vi "set_status_string.vi"(8 "error in":errorcluster, 9 "new line?":bool=TRUE, 10 "status string in":string, 11 "controls array":refnum<vi>[](array[refnum])) -> (0 "error out":errorcluster, 3 "controls array out":refnum<vi>[](array[refnum]))   [LabVIEW 2019]
panel:
  out "output string":string
  # "SET STATUS STRING"
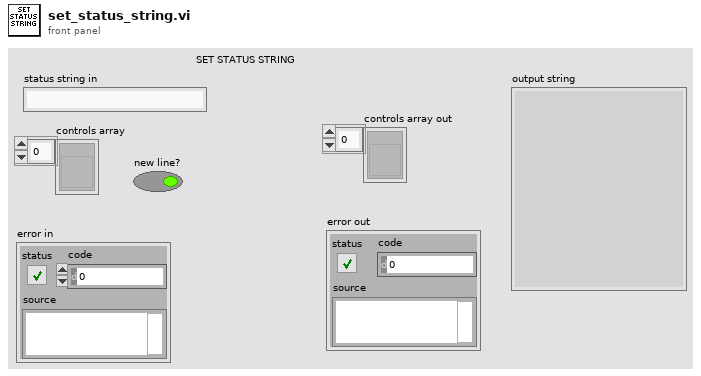
[diagram p1: front panel]
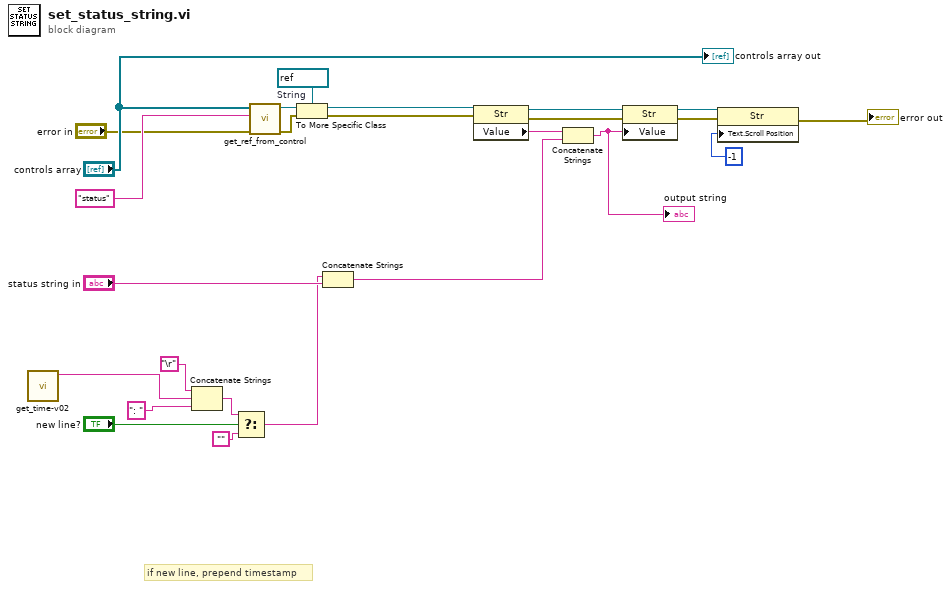
[diagram p0: block diagram]
diagram:
  w22 = refnum<vi> refnum  # String
  # "if new line, prepend timestamp"
  n1 = call "get_time-v02.vi"() -> ("pure text output"=w11:string)  [unwired: 10 in, 1 out]
  n2 = Concatenate Strings("\r", w11, ": " ("string")) -> (w8:string)
  n3 = Select(t=w8, s="new line?", f="") -> (s? t:f=w7:string)
  n4 = call "get_ref_from_control.vi"("error in"="error in", "control label"="status", "controls array"="controls array") -> ("error out"=w21:errorcluster, "reference out"=w23:refnum<vi>)  [unwired: 7 in]
  n5 = To More Specific Class(target class=w22, reference=w23, error in=w21) -> (specific class reference=w5:refnum<vi>, error out=w4:errorcluster)
  n6 = Concatenate Strings(w7, "status string in") -> (w14:string)
  n7 = property class="Str"(reference=w5, error in=w4) -> (reference out=w19:refnum<vi>, error out=w20:errorcluster, "Value"=w16:string)
  n8 = Concatenate Strings(w16, w14) -> (w15:string)
  "output string" <- w15
  n9 = property class="Str"(reference=w19, error in=w20, "Value"=w15) -> (reference out=w3:refnum<vi>, error out=w2:errorcluster)
  n10 = property class="Str"(reference=w3, error in=w2, "Text.Scroll Position"=-1) -> (error out=→"error out":errorcluster)  [unwired: 1 out]
  "controls array out" <- "controls array"
